vi "get_control_refs.vi"(8 "error in (no error)":errorcluster, 11 "ImagingModeDL090130Frame in":refnum<class "ImagingModeDL090130Frame.lvclass">) -> (0 "error out":errorcluster, 2 "control refs":T1, 3 "ImagingModeDL090130Frame out":refnum<class "ImagingModeDL090130Frame.lvclass">)   [LabVIEW 2010, in "ImagingModeDL090130Frame.lvclass"]
uses:
  ImagingModeDL090130Frame.lvclass
  control_refs.ctl
  common/xcontrols/XIntensityCompensation/XIntensityCompensation/XIntensityCompensation.xctl
  class_data.vi
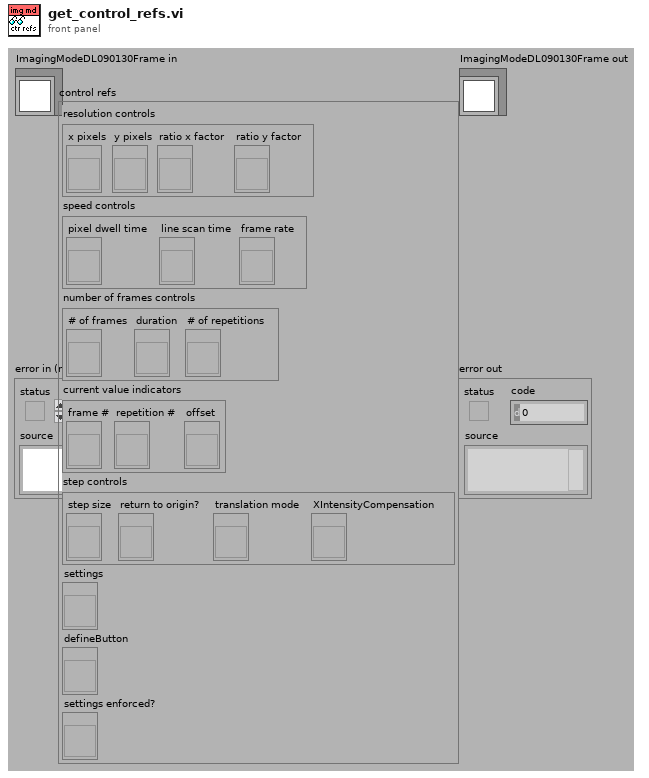
[diagram p1: front panel]
types:
  T1 = typedef "ImagingModeDL090130Frame.lvclass/control_refs.ctl" = cluster{"resolution controls":cluster{"x pixels":refnum<vi>, "y pixels":refnum<vi>, "ratio x factor":refnum<vi>, "ratio y factor":refnum<vi>}, "speed controls":cluster{"pixel dwell time":refnum<vi>, "line scan time":refnum<vi>, "frame rate":refnum<vi>}, "number of frames controls":cluster{"# of frames":refnum<vi>, "duration":refnum<vi>, "# of repetitions":refnum<vi>}, "current value indicators":cluster{"frame #":refnum<vi>, "repetition #":refnum<vi>, "offset":refnum<vi>}, "step controls":cluster{"step size":refnum<vi>, "return to origin?":refnum<vi>, "translation mode":refnum<vi>, "XIntensityCompensation":refnum<vi>}, "settings":refnum<vi>, "defineButton":refnum<vi>, "settings enforced?":refnum<vi>}
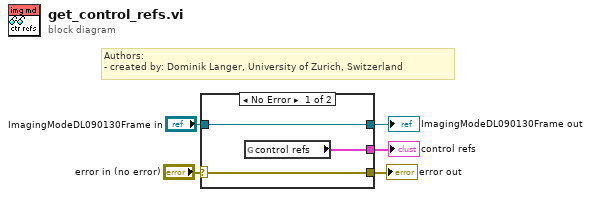
[diagram p0: block diagram]
diagram:
  # "Authors: \n- created by: Dominik Langer, University of Zurich, Switzerland"
  n1 = case shown="No Error" "error in (no error)" {
    selector: "error in (no error)" -> [w7 w10]
    tunnel: [w7 w10] -> w4
    tunnel: [w8 w9] -> w2
    tunnel: "ImagingModeDL090130Frame in" -> [w8 w9]
    tunnel: [w6 _] -> w1
    frame No Error {
      n2 = global read "class_data.vi" "control refs"() -> (w6:T1)
    }
    frame Error {
    }
  }
  "error out" <- w4
  "ImagingModeDL090130Frame out" <- w2
  "control refs" <- w1
